vi "Item_OnPopupMenu.vi"(11 "Object":T1) -> ()   [LabVIEW 2018, in "LVClassByRef.lvlib"]
uses:
  <resource>/Framework/Providers/LVClassByRef/LVClassByRef.lvlib
  <resource>/Framework/Providers/API/ItemRef.ctl
  <resource>/Framework/Providers/API/mxLvMenuItem.ctl
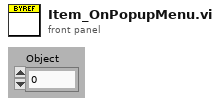
[diagram p1: front panel]
types:
  T1 = typedef "ItemRef.ctl" = u64
  T2 = typedef "mxLvMenuItem.ctl" = cluster{"Menu Name":string, "Description":string, "Icon File Name":path, "Menu Tag":string, "Enabled":bool, "Checked":bool, "Separator":bool, "Batchable":bool, "Weight":i32, "Batch Mode (Ignored if Not Batchable)":enum32{"Show If All Items Support Command", "Show If Any Items Support Command"}, "Menu Location":enum32{"<None>", "Project", "Project / Build Specifications", "Tools", "Tools / Source Control", "Tools / Real-Time Module", "Help"}, "Exclude From Getting Started Window Menu":bool}
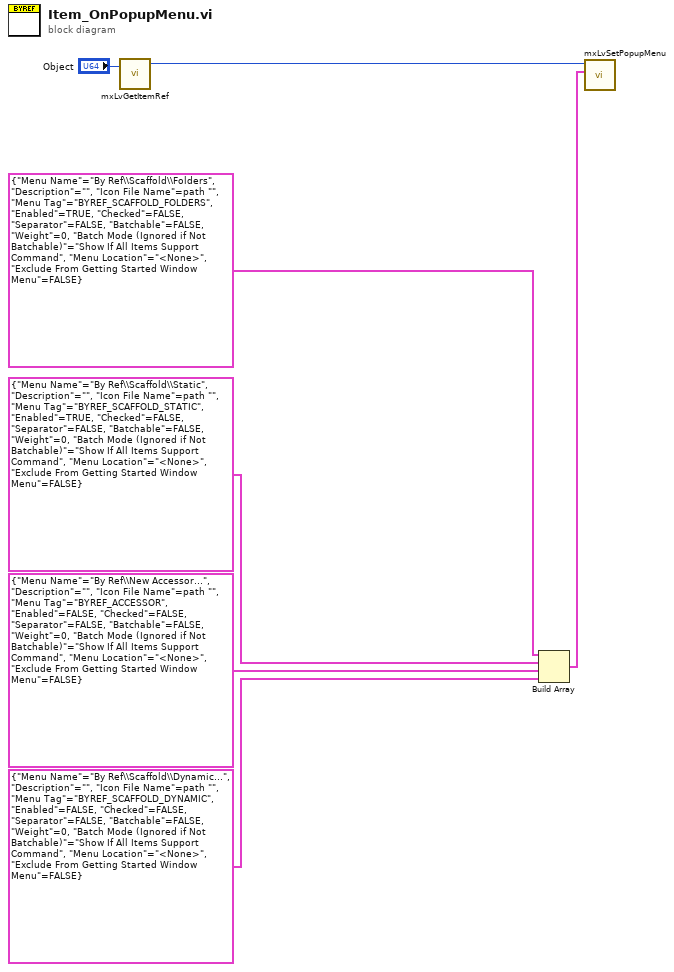
[diagram p0: block diagram]
diagram:
  n1 = call <resource>:"mxLvGetItemRef.vi"("Item"="Object") -> ("Item"=w5:T1)  [unwired: 1 in, 2 out]
  n2 = Build Array(T2 {"Menu Name"="By Ref\\Scaffold\\Folders", "Description"="", "Icon File Name"=path "", "Menu Tag"="BYREF_SCAFFOLD_FOLDERS", "Enabled"=TRUE, "Checked"=FALSE, "Separator"=FALSE, "Batchable"=FALSE, "Weight"=0, "Batch Mode (Ignored if Not Batchable)"=enum."Show If All Items Support Command", "Menu Location"=enum."<None>", "Exclude From Getting Started Window Menu"=FALSE} ("Menu Item"), T2 {"Menu Name"="By Ref\\Scaffold\\Static", "Description"="", "Icon File Name"=path "", "Menu Tag"="BYREF_SCAFFOLD_STATIC", "Enabled"=TRUE, "Checked"=FALSE, "Separator"=FALSE, "Batchable"=FALSE, "Weight"=0, "Batch Mode (Ignored if Not Batchable)"=enum."Show If All Items Support Command", "Menu Location"=enum."<None>", "Exclude From Getting Started Window Menu"=FALSE} ("Menu Item"), T2 {"Menu Name"="By Ref\\New Accessor...", "Description"="", "Icon File Name"=path "", "Menu Tag"="BYREF_ACCESSOR", "Enabled"=FALSE, "Checked"=FALSE, "Separator"=FALSE, "Batchable"=FALSE, "Weight"=0, "Batch Mode (Ignored if Not Batchable)"=enum."Show If All Items Support Command", "Menu Location"=enum."<None>", "Exclude From Getting Started Window Menu"=FALSE} ("Menu Item"), T2 {"Menu Name"="By Ref\\Scaffold\\Dynamic...", "Description"="", "Icon File Name"=path "", "Menu Tag"="BYREF_SCAFFOLD_DYNAMIC", "Enabled"=FALSE, "Checked"=FALSE, "Separator"=FALSE, "Batchable"=FALSE, "Weight"=0, "Batch Mode (Ignored if Not Batchable)"=enum."Show If All Items Support Command", "Menu Location"=enum."<None>", "Exclude From Getting Started Window Menu"=FALSE} ("Menu Item")) -> (w7:T2[])
  n3 = call <resource>:"mxLvSetPopupMenu.vi"("Popup Menu Items"=w7, "Item"=w5) -> ()  [unwired: 8 in, 2 out]
